vi "Digital Read Pulse Width.vi"(5 "Stimulus Pulse (Active High)":T2=enum."Active High", 6 "Timeout  (250 mS)":u32=250, 7 "Incoming Pulse Polarity (Active High)":T1=enum."Active High", 8 "Error In":errorcluster, 9 "DO Channel":u8, 10 "DI Channel":u8, 11 "LINX Resource":T3) -> (0 "Error Out":errorcluster, 2 "Pulse Width (uS)":u32, 3 "LINX Resource":T3)   [LabVIEW 2013, in "LVH-LINX.lvlib"]
doc: "Read a digital pulse width. Use the Stimulus input to specify a pulse type to send before measuring the response pulse."
uses:
  LVH-LINX.lvlib
  Private/Type Defs/LINX Ref.ctl
  Private/Type Defs/Platform.ctl
  Private/Type Defs/Interface.ctl
  Private/Device/Type Defs/LINX Device Config.ctl
  Private/Device/Type Defs/TCP Config.ctl
  Private/Type Defs/Device Family.ctl
  Private/Device/Type Defs/Channels.ctl
  Private/Device/Type Defs/Stimulus Pulse.ctl
  Private/Device/Type Defs/Pulse Polarity.ctl
  Private/Type Defs/Peripheral.ctl
  Private/Type Defs/Error Type.ctl
  Private/Device/Device.lvlib
  Private/myRIO/myRIO.lvlib
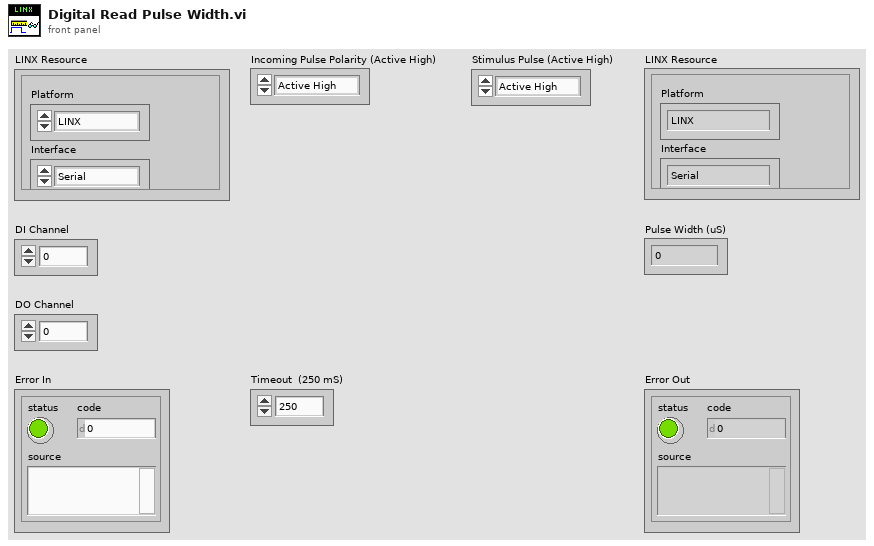
[diagram p1: front panel]
types:
  T1 = typedef "LVH-LINX.lvlib/Device.lvlib/Pulse Polarity.ctl" = enum8{"Active Low", "Active High"}
  T2 = typedef "LVH-LINX.lvlib/Device.lvlib/Stimulus Pulse.ctl" = enum16{"None", "Active Low", "Active High"}
  T3 = typedef "LVH-LINX.lvlib/LINX Ref.ctl" = cluster{"Platform":T4, "Interface":T5, "LINX Device Config":T6}
  T4 = typedef "LVH-LINX.lvlib/Platform.ctl" = enum16{"LINX", "myRIO"}
  T5 = typedef "LVH-LINX.lvlib/Interface.ctl" = enum16{"Serial", "TCP"}
  T6 = typedef "LVH-LINX.lvlib/Device.lvlib/LINX Device Config.ctl" = cluster{"Interface":T5, "COM Port":refnum<visa-resource-name>, "TCP Configuration":T7, "Device Family":T8, "Device ID":u8, "Device Name":string, "TCP Ref":refnum<k5>, "Channels":T9}
  T7 = typedef "LVH-LINX.lvlib/Device.lvlib/TCP Config.ctl" = cluster{"IP Address":string, "Port":u16}
  T8 = typedef "LVH-LINX.lvlib/Device Family.ctl" = enum8{"National Instruments", "Digilent", "Arduino"}
  T9 = typedef "LVH-LINX.lvlib/Channels.ctl" = cluster{"DI Channels":u8[], "DO Channels":u8[], "AI":u8[], "AO":u8[], "PWM":u8[], "QE":u8[], "UART":u8[], "I2C 2":u8[], "SPI":u8[], "CAN":u8[], "AI Ref (V)":dbl, "AO Resolution (Bits)":u8, "AO Ref (V)":dbl}
  T10 = typedef "LVH-LINX.lvlib/Peripheral.ctl" = enum8{"DI", "DO", "AI", "AO", "PWM", "QE", "UART", "I2C", "SPI", "CAN"}
  T11 = typedef "LVH-LINX.lvlib/Error Type.ctl" = enum16{"Unknown", "Timeout", "Corrupt Return Packet", "Unable To Connect", "Command Not Supported", "Channel DNE", "Invalid COM Config", "Firmware Version Mismatch"}
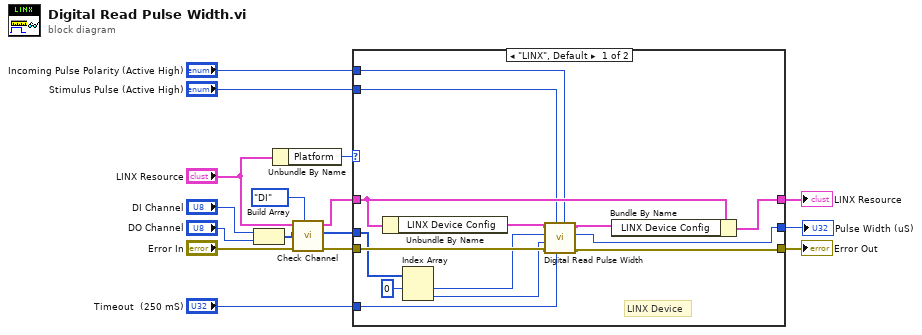
[diagram p0: block diagram]
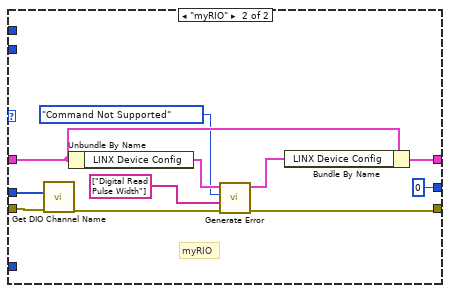
[diagram p2: hidden frame]
diagram:
  n1 = Build Array("DI Channel", "DO Channel") -> (w6:u8[])
  n2 = Unbundle By Name("LINX Resource") -> ("Platform"=w16:T4)
  n3 = call "Check Channel.vi"("Peripheral"=Peripheral."DI", "Error In"="Error In", "Channels"=w6, "LINX Resource"="LINX Resource") -> ("Error Out"=w13:errorcluster, "Channels"=w12:u8[], "LINX Resource"=w10:T3)  [unwired: 5 in]
  n4 = case shown="\"LINX\", Default" w16 {
    tunnel: w13 -> [w26 w41]
    tunnel: w10 -> [w30 w34]
    tunnel: [w25 w38] -> w15
    tunnel: [w29 w35] -> w14
    tunnel: w12 -> [w24 w40]
    tunnel: [w21 u32 0 ("Pulse Width (uS)")] -> w5
    tunnel: "Incoming Pulse Polarity (Active High)" -> [w19 _]
    tunnel: "Stimulus Pulse (Active High)" -> [w20 _]
    tunnel: "Timeout  (250 mS)" -> [w18 _]
    frame "LINX", Default {
      # "LINX Device"
      n5 = Unbundle By Name(w30) -> ("LINX Device Config"=w27:T6)
      n6 = Index Array(array=w24, index #1=0 ("index")) -> (element #1=w22:u8, element #2=w17:u8)  [unwired: 1 in]
      n7 = call "Digital Read Pulse Width.vi"("Incoming Pulse Polarity (Active High)"=w19, "Timeout  (250 mS)"=w18, "Stimulus Pulse (Active High)"=w20, "Error In"=w26, "DO Channel (0)"=w17, "DI Channel (0)"=w22, "LINX Device Config"=w27) -> ("Error Out"=w25:errorcluster, "Pulse Width (uS)"=w21:u32, "LINX Device Config"=w28:T6)  [unwired: 2 in]
      n8 = Bundle By Name(cluster=w30, "LINX Device Config"=w28) -> (w29:T3)
    }
    frame "myRIO" {
      # "myRIO"
      n9 = call "Get DIO Channel Name.vi"("Error In"=w41, "DIO Channel Nums"=w40) -> ("Error Out"=w39:errorcluster)  [unwired: 8 in, 1 out]
      n10 = Unbundle By Name(w34) -> ("LINX Device Config"=w36:T6)
      n11 = call "Generate Error.vi"("Error In"=w39, "Arguments"=string[] ["Digital Read Pulse Width"], "Error Type"=Error_Type."Command Not Supported", "LINX Device Config"=w36) -> ("Error Out"=w38:errorcluster, "LINX Device Config"=w37:T6)  [unwired: 6 in]
      n12 = Bundle By Name(cluster=w34, "LINX Device Config"=w37) -> (w35:T3)
    }
  }
  "Error Out" <- w15
  "LINX Resource" <- w14
  "Pulse Width (uS)" <- w5
